vi "SimpleWizard.vi"() -> ()   [LabVIEW 2016]
panel:
  out "Console Out":string
  out "new picture":picture
  out "Version":string
  in  "stop":bool
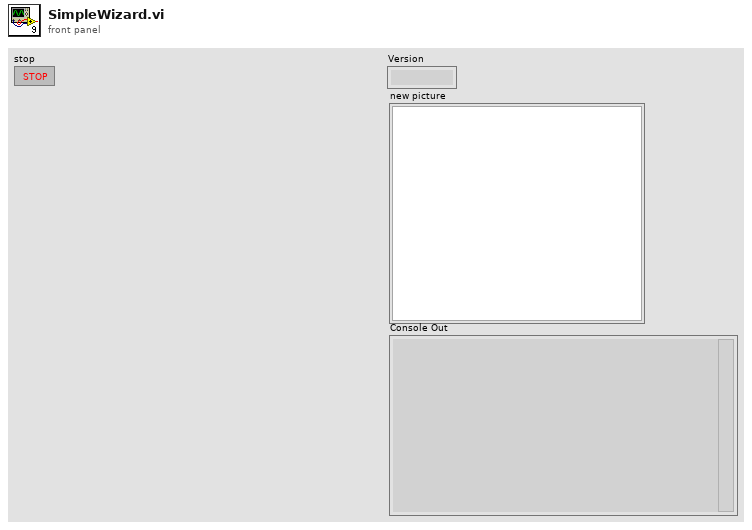
[diagram p1: front panel]
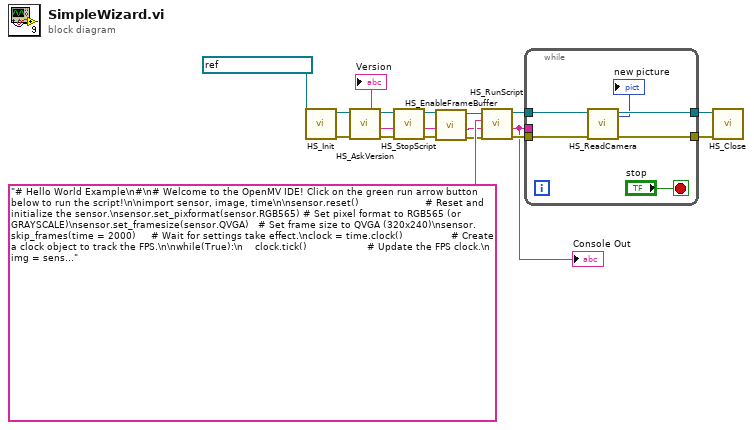
[diagram p0: block diagram]
diagram:
  n1 = call "HS_Init.vi"("VISA Refnum in"=refnum<visa-resource-name> "ASRL12::INSTR") -> ("error out"=w19:errorcluster, "VISA Refnum out"=w18:refnum<visa-resource-name>)  [unwired: 9 in]
  n2 = call "HS_AskVersion.vi"("error in"=w19, "VISA Refnum in"=w18) -> ("error out"=w10:errorcluster, "Console Out"=w9:string, "Version"=→"Version":string, "VISA Refnum out"=w8:refnum<visa-resource-name>)  [unwired: 6 in]
  n3 = call "HS_StopScript.vi"("error in"=w10, "Console In"=w9, "VISA Refnum in"=w8) -> ("error out"=w7:errorcluster, "Console Out"=w6:string, "VISA Refnum out"=w5:refnum<visa-resource-name>)  [unwired: 5 in, 1 out]
  n4 = call "HS_EnableFrameBuffer.vi"("error in"=w7, "Console In"=w6, "VISA Refnum in"=w5) -> ("error out"=w4:errorcluster, "Console Out"=w2:string, "VISA Refnum out"=w3:refnum<visa-resource-name>)  [unwired: 5 in, 1 out]
  n5 = call "HS_RunScript.vi"("error in"=w4, "Console In"=w2, "script"="# Hello World Example\n#\n# Welcome to the OpenMV IDE! Click on the green run arrow button below to run the script!\n\nimport sensor, image, time\n\nsensor.reset()                      # Reset and initialize the sensor.\nsensor.set_pixformat(sensor.RGB565) # Set pixel format to RGB565 (or GRAYSCALE)\nsensor.set_framesize(sensor.QVGA)   # Set frame size to QVGA (320x240)\nsensor.skip_frames(time = 2000)     # Wait for settings take effect.\nclock = time.clock()                # Create a clock object to track the FPS.\n\nwhile(True):\n    clock.tick()                    # Update the FPS clock.\n    img = sensor.snapshot()         # Take a picture and return the image.\n#    print(clock.fps())              # Note: OpenMV Cam runs about half as fast when connected\n                                    # to the IDE. The FPS should increase once disconnected.\n", "VISA Refnum in"=w3) -> ("error out"=w13:errorcluster, "Console Out"=w1:string, "VISA Refnum out"=w14:refnum<visa-resource-name>)  [unwired: 4 in, 1 out]
  "Console Out" <- w1
  n6 = while {
    tunnel: w14 -> [w24]
    tunnel: w13 -> [w22]
    tunnel: [w21] -> w12
    tunnel: [w23] -> w11
    tunnel: w1 -> [_]
    stop <- "stop" stop-if-true
    n7 = call "HS_ReadCamera.vi"("error in"=w22, "VISA Refnum in"=w24) -> ("error out"=w21:errorcluster, "VISA Refnum out"=w23:refnum<visa-resource-name>, "new picture"=→"new picture":picture)  [unwired: 2 in, 5 out]
  }
  n8 = call "HS_Close.vi"("error in (no error)"=w12, "VISA Refnum in"=w11) -> ()  [unwired: 10 in]
